vi "GetImages.vi"(4 "File type":T1, 5 "Disabled":bool, 6 "Background Color":u32(colorbox), 7 "image directory":path, 8 "error in":errorcluster, 11 "Control in":refnum<class "Control.lvclass">) -> (0 "error out":errorcluster, 3 "Control out":refnum<class "Control.lvclass">)   [LabVIEW 2014, in "Raspberry Pi Compatible Compiler for LabVIEW.lvlib" / "Control.lvclass"]
uses:
  Control.lvclass
  ImageTypes.ctl
  Raspberry Pi Compatible Compiler for LabVIEW.lvlib
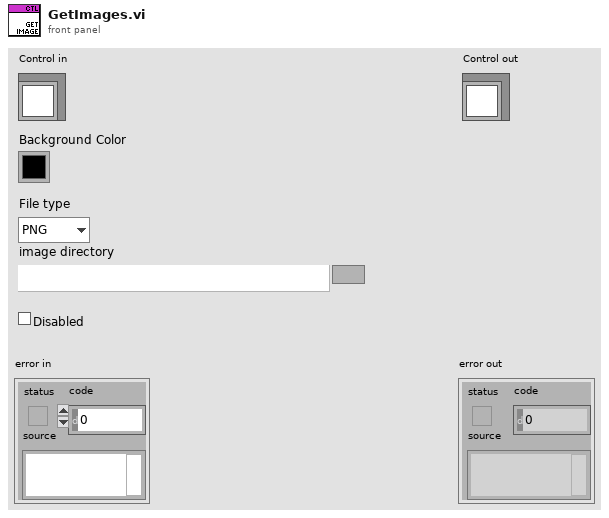
[diagram p1: front panel]
types:
  T1 = typedef "Raspberry Pi Compatible Compiler for LabVIEW.lvlib/ImageTypes.ctl" = enum16{"PNG", "JPEG", "BMP"}
  T2 = typedef "imagedata.ctl" = cluster{"image type":i32, "image depth":i32, "image":u8[], "mask":u8[], "colors":u32[], "Rectangle":cluster{"left":i16, "top":i16, "right":i16, "bottom":i16}}
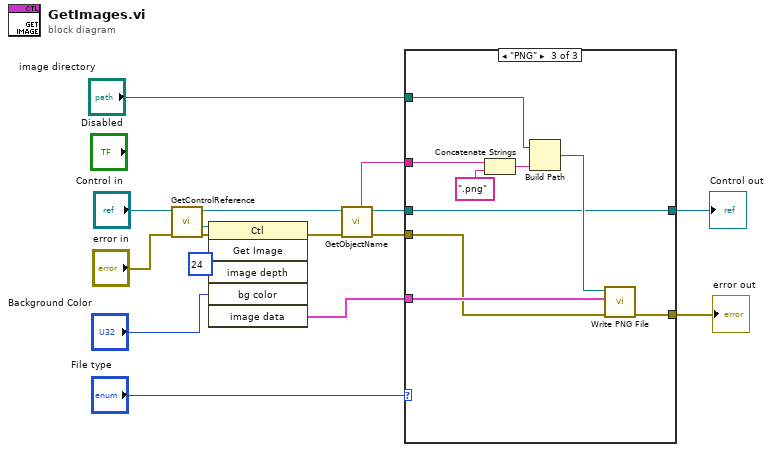
[diagram p0: block diagram]
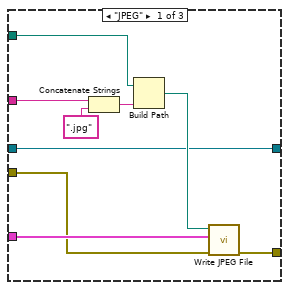
[diagram p2: hidden frame]
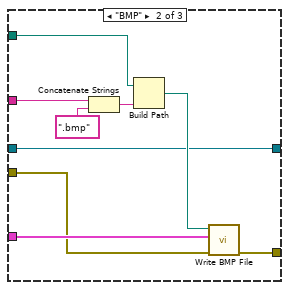
[diagram p3: hidden frame]
diagram:
  n1 = call "GetControlReference.vi"("error in"="error in", "Control in"="Control in") -> ("error out"=w12:errorcluster, "control reference"=w13:refnum<vi>, "Control out"=w8:refnum<class "Control.lvclass">)  [unwired: 7 in]
  n2 = invoke class="Ctl" method="Get Image"(reference=w13, error in=w12, "image depth"=24 ("Image Depth"), "bg color"="Background Color") -> (error out=w7:errorcluster, "image data"=w9:T2)  [unwired: 2 in, 4 out]
  n3 = call-dynamic "GetObjectName.vi"("error in"=w7, "GObject in"=w8) -> ("error out"=w6:errorcluster, "GObject out"=w5:refnum<class "Control.lvclass">, "Name"=w4:string)  [unwired: 5 in]
  n4 = case shown="\"PNG\"" "File type" {
    tunnel: w9 -> [w25 w34 w43]
    tunnel: [w24 w33 w42] -> w1
    tunnel: w6 -> [w23 w32 w41]
    tunnel: w5 -> [w17 w26 w35]
    tunnel: w4 -> [w22 w31 w40]
    tunnel: "image directory" -> [w19 w28 w37]
    tunnel: [w17 w26 w35] -> w2
    frame "JPEG" {
      n5 = Concatenate Strings(w22, ".jpg" ("string")) -> (w20:string)
      n6 = Build Path(base path=w19, name or relative path=w20) -> (appended path=w18:path)
      n7 = call <vilib>:"Write JPEG File.vi"("error in (no error)"=w23, "image data"=w25, "path to JPEG file"=w18) -> ("error out"=w24:errorcluster)  [unwired: 7 in, 1 out]
    }
    frame "BMP" {
      n8 = Concatenate Strings(w31, ".bmp" ("string")) -> (w29:string)
      n9 = Build Path(base path=w28, name or relative path=w29) -> (appended path=w27:path)
      n10 = call <vilib>:"Write BMP File.vi"("error in (no error)"=w32, "image data"=w34, "path to BMP file"=w27) -> ("error out"=w33:errorcluster)  [unwired: 7 in, 1 out]
    }
    frame "PNG" {
      n11 = Concatenate Strings(w40, ".png" ("string")) -> (w38:string)
      n12 = Build Path(base path=w37, name or relative path=w38) -> (appended path=w36:path)
      n13 = call <vilib>:"Write PNG File.vi"("error in (no error)"=w41, "image data"=w43, "path to PNG file"=w36) -> ("error out"=w42:errorcluster)  [unwired: 7 in, 1 out]
    }
  }
  "error out" <- w1
  "Control out" <- w2
